vi "Main.vi"() -> ()   [LabVIEW 2020]
uses:
  <vilib>/Instr/_visa.llb/VISA Configure Serial Port (Instr).vi
panel:
  out "布尔":bool
  in  "帮助":bool
  in  "发送信息":bool
  in  "定时周期":dbl=1000.0 caption="周期："
  in  "发送新行":bool
  in  "定时发送":bool
  in  "发送信息":string
  in  "清除发送信息":bool
  in  "清除接收信息":bool
  out "接收信息":string
  out "状态指示灯":bool
  in  "串口操作":bool
  in  "停止位":u16(ring)=10 caption="停止位（10: 1位）" items=["1.0"=10, "1.5"=15, "2.0"=20]
  in  "数据位":u16(ring)=8 items=["8"=8, "7"=7, "6"=6, "5"=5]
  in  "检验位":enum16{"None", "Odd", "Even", "Mark", "Space"}(ring) caption="奇偶（0:无）"
  in  "波特率":u32(ring)=9600 items=["110"=110, "300"=300, "600"=600, "1200"=1200, "2400"=2400, "4800"=4800, "9600"=9600, "14400"=14400, "19200"=19200, "38400"=38400, "43000"=43000, "57600"=57600, "76800"=76800, "115200"=115200, "128000"=128000, "230400"=230400, "256000"=256000, "460800"=460800, "921600"=921600, "1000000"=1000000, "2000000"=2000000, "3000000"=3000000]
  in  "VISA资源名称":refnum<visa-resource-name>="COM1" caption="串口选择"
  in  "停止":bool
  # "ms"
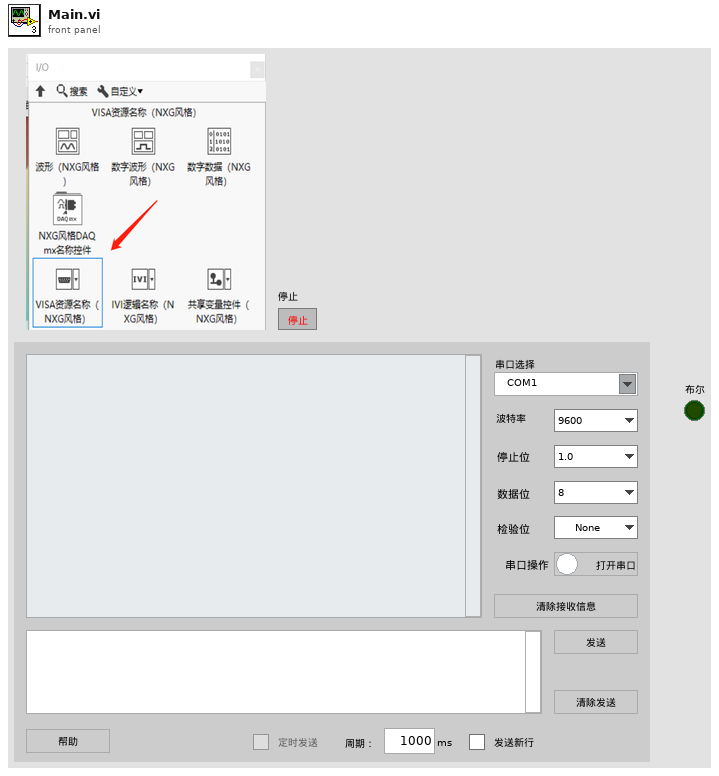
[diagram p1: front panel]
types:
  T1 = enum8{"Enabled", "Disabled", "Disabled and Grayed Out"}
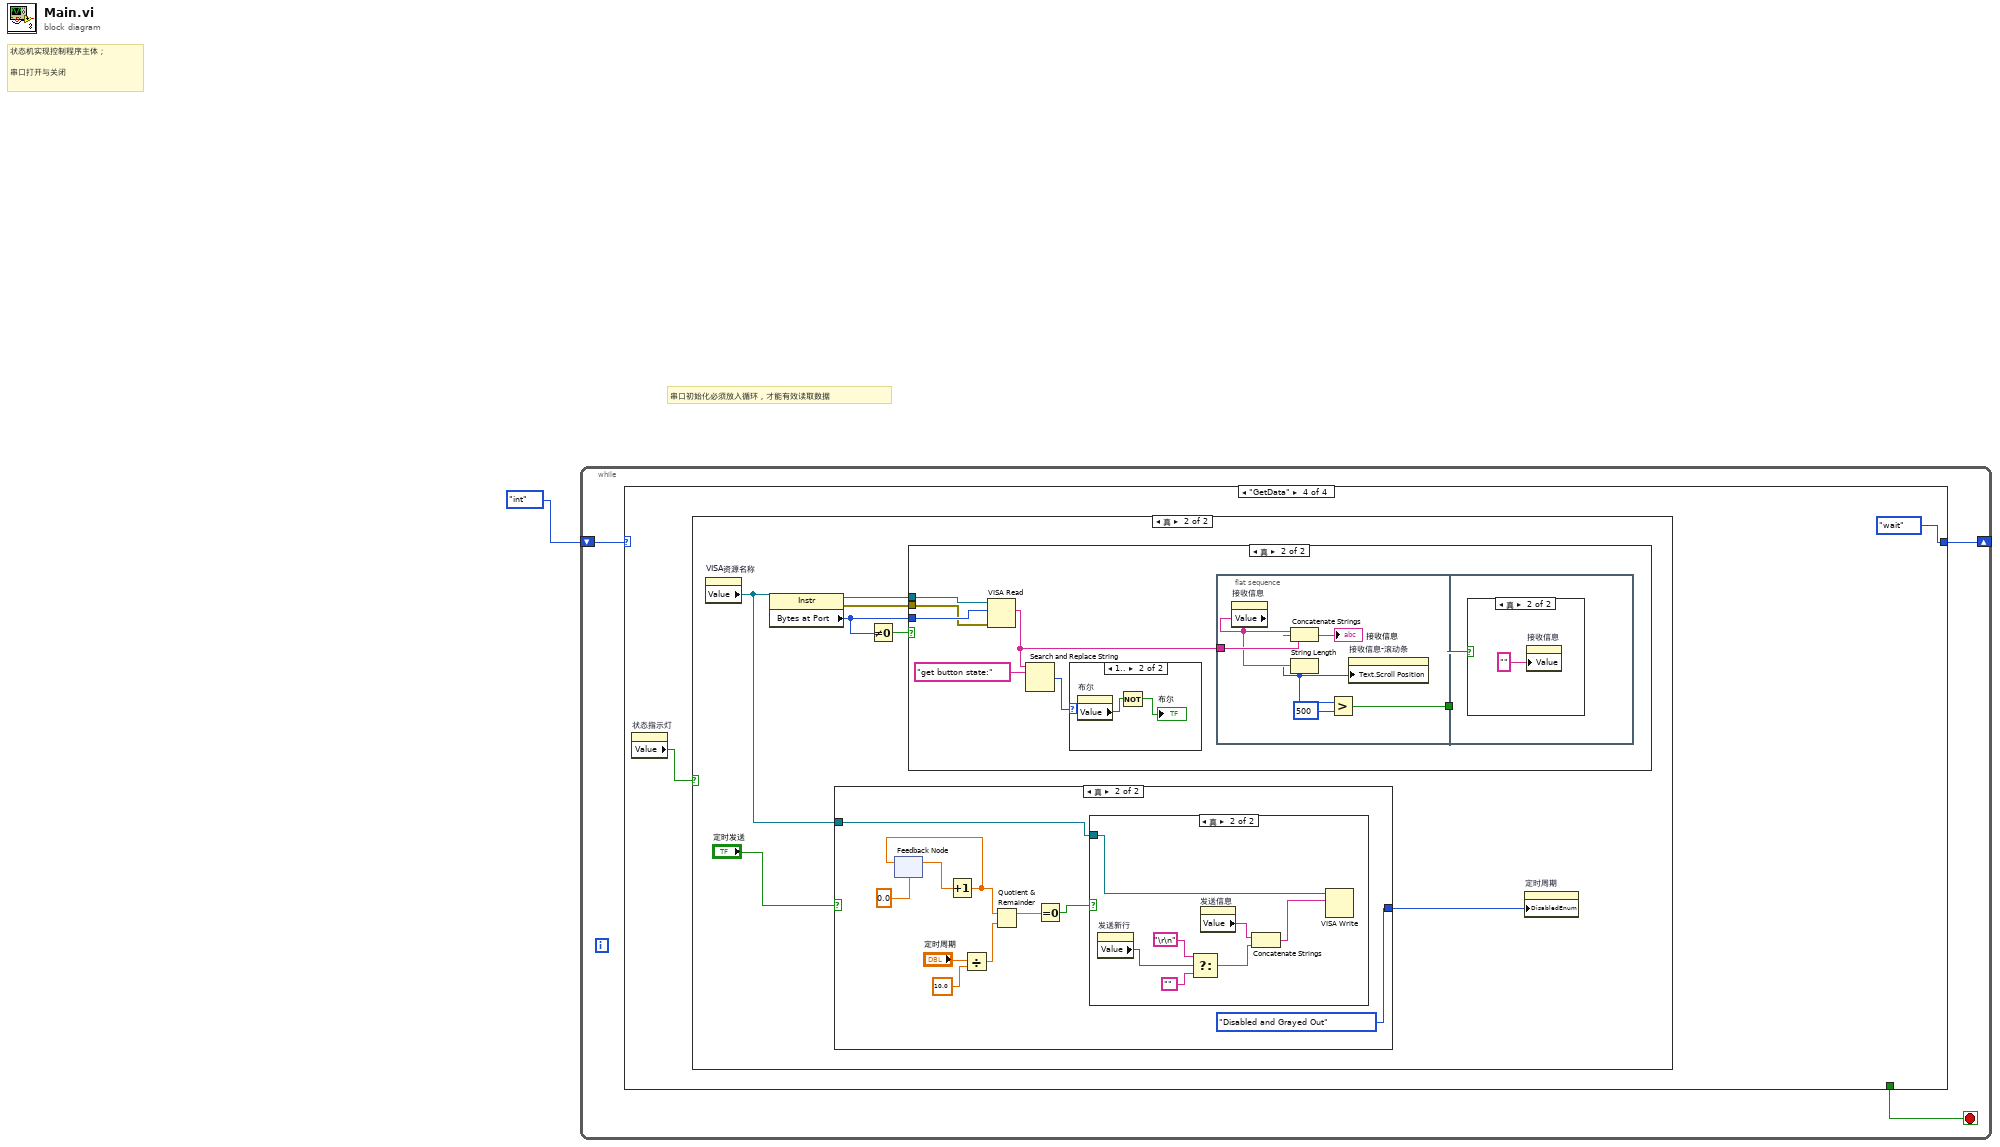
[diagram p0: block diagram]
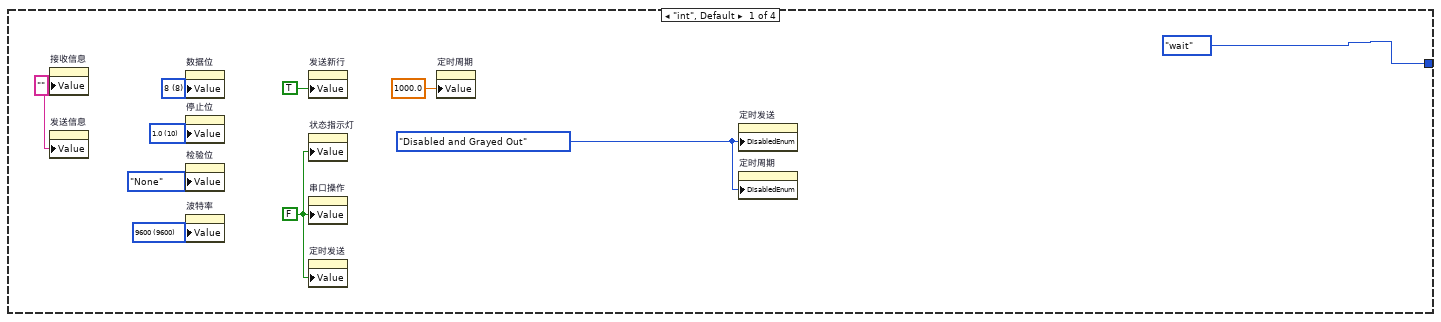
[diagram p2: hidden frame]
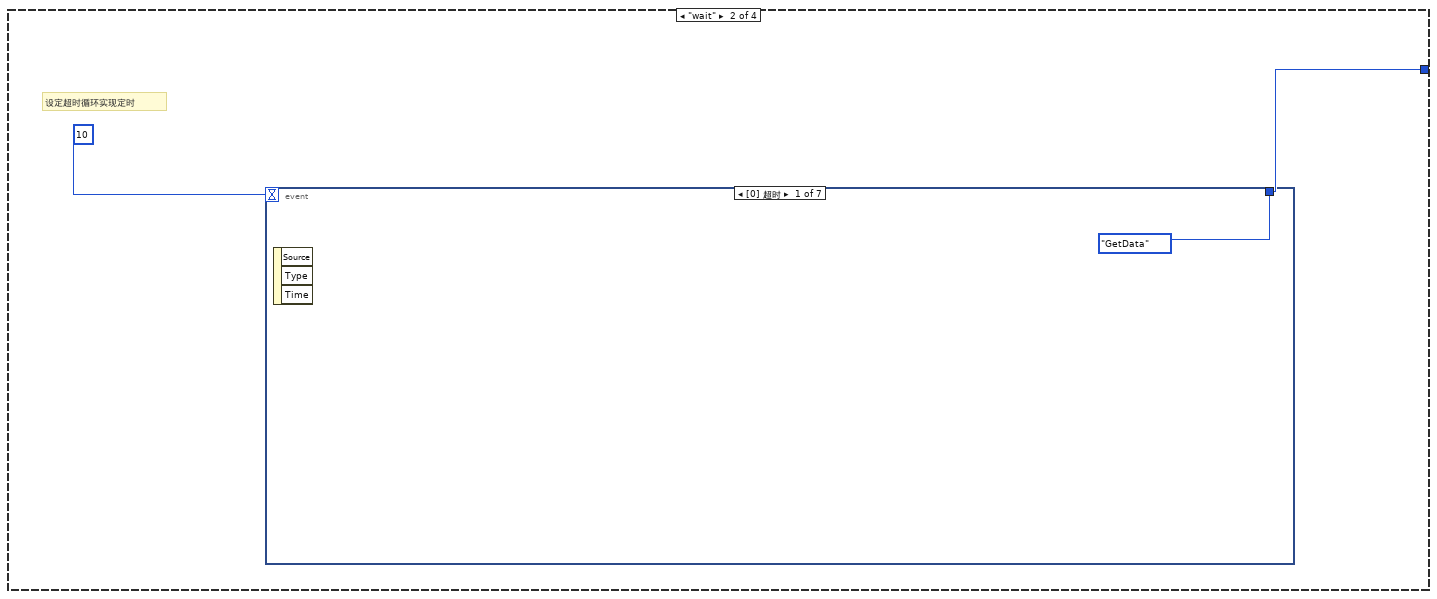
[diagram p3: hidden frame]
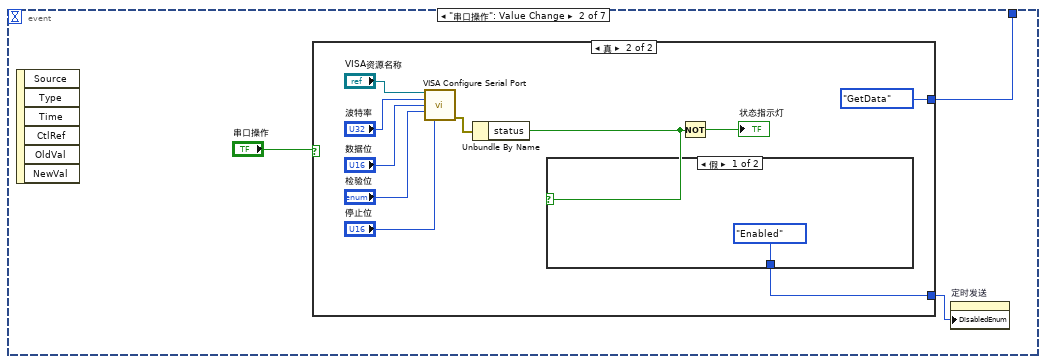
[diagram p4: hidden frame]
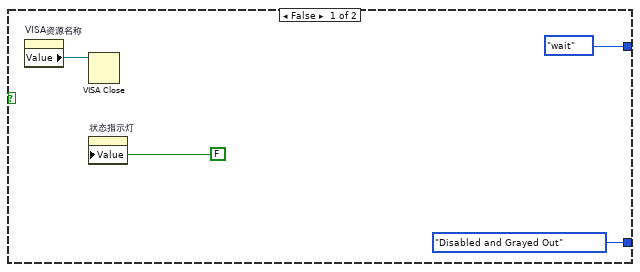
[diagram p5: hidden frame]
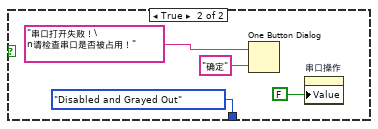
[diagram p6: hidden frame]
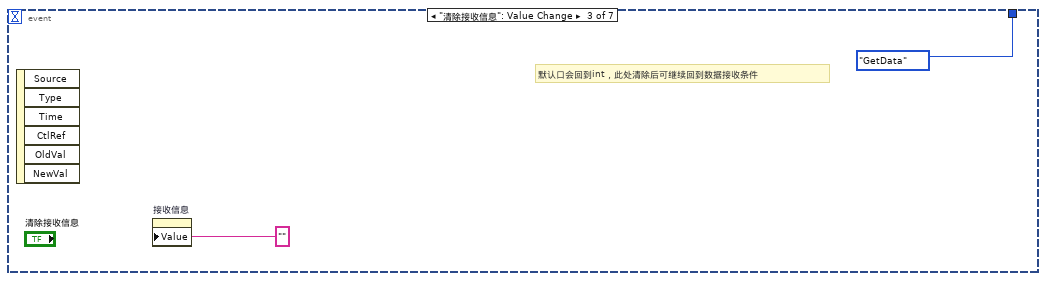
[diagram p7: hidden frame]
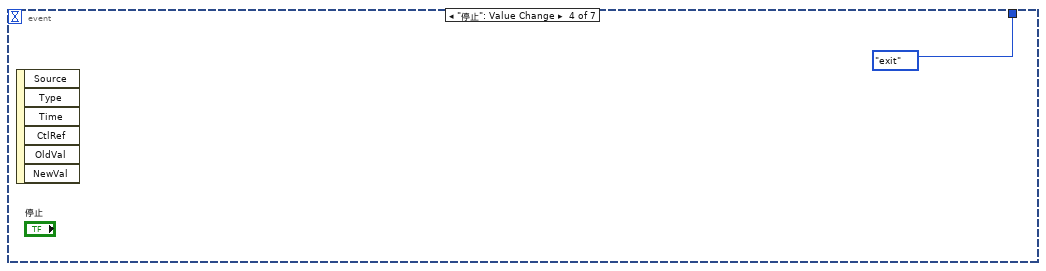
[diagram p8: hidden frame]
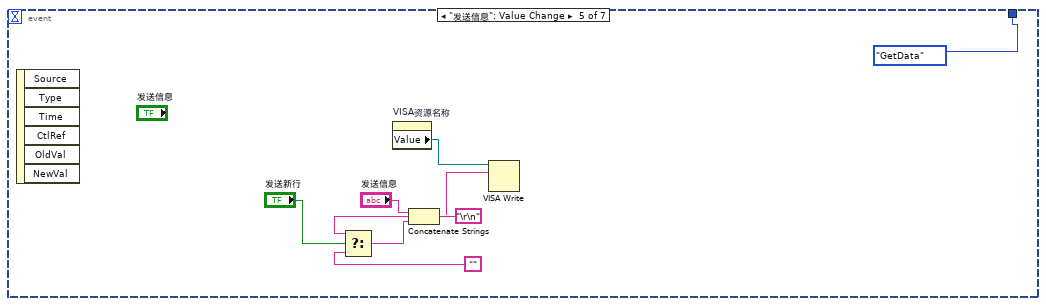
[diagram p9: hidden frame]
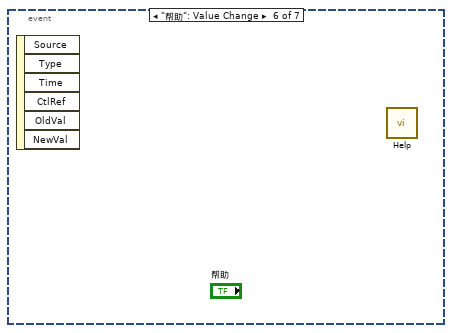
[diagram p10: hidden frame]
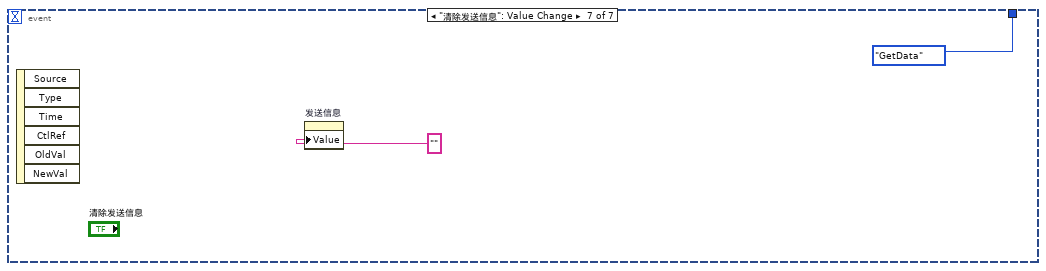
[diagram p11: hidden frame]
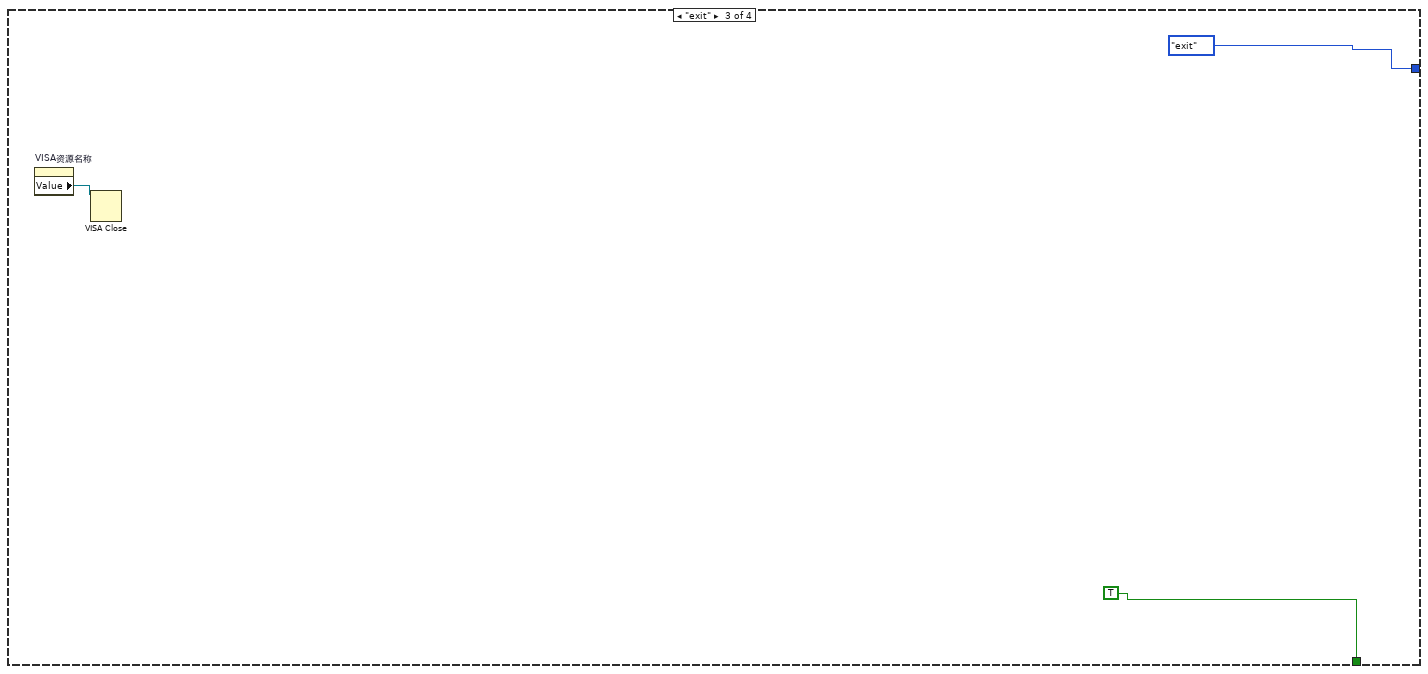
[diagram p12: hidden frame]
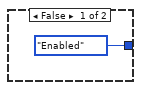
[diagram p14: hidden frame]
diagram:
  # "串口初始化必须放入循环，才能有效读取数据"
  # "状态机实现控制程序主体；\n\n串口打开与关闭"
  n1 = while {
    shift-right: [w3] -> _
    shift-left: enum16{"int", "wait", "exit", "GetData"}."int" -> [w4]
    stop <- w2 stop-if-true
    n2 = case shown="\"GetData\"" w4 {
      tunnel: [enum16{"int", "wait", "exit", "GetData"}."wait" w15 enum16{"int", "wait", "exit", "GetData"}."exit" enum16{"int", "wait", "exit", "GetData"}."wait"] -> w3
      tunnel: [_ _ TRUE _] -> w2
      frame "int", Default {
        w5 = T1."Disabled and Grayed Out" ("禁用")
        w6 = FALSE ("状态指示灯")
        w11 = u32 9600 items=["110"=110, "300"=300, "600"=600, "1200"=1200, "2400"=2400, "4800"=4800, "9600"=9600, "14400"=14400, "19200"=19200, "38400"=38400, "43000"=43000, "57600"=57600, "76800"=76800, "115200"=115200, "128000"=128000, "230400"=230400, "256000"=256000, "460800"=460800, "921600"=921600, "1000000"=1000000, "2000000"=2000000, "3000000"=3000000] ("波特率")
        w12 = u16 8 items=["8"=8, "7"=7, "6"=6, "5"=5] ("数据位")
        w13 = u16 10 items=["1.0"=10, "1.5"=15, "2.0"=20] ("停止位")
        w8 = "" ("接收信息")
        n3 = property on="接收信息" class="Str"("Value"=w8) -> ()  [unwired: 2 in, 2 out]
        n4 = property on="发送信息" class="Str"("Value"=w8) -> ()  [unwired: 2 in, 2 out]
        n5 = property on="数据位" class="Ring (严格)"("Value"=w12) -> ()  [unwired: 2 in, 2 out]
        n6 = property on="停止位" class="Ring (严格)"("Value"=w13) -> ()  [unwired: 2 in, 2 out]
        n7 = property on="检验位" class="Enum (严格)"("Value"=enum16{"None", "Odd", "Even", "Mark", "Space"}."None" ("检验位")) -> ()  [unwired: 2 in, 2 out]
        n8 = property on="波特率" class="Ring (严格)"("Value"=w11) -> ()  [unwired: 2 in, 2 out]
        n9 = property on="发送新行" class="Bool (严格)"("Value"=TRUE ("发送新行")) -> ()  [unwired: 2 in, 2 out]
        n10 = property on="状态指示灯" class="Bool (严格)"("Value"=w6) -> ()  [unwired: 2 in, 2 out]
        n11 = property on="串口操作" class="Bool (严格)"("Value"=w6) -> ()  [unwired: 2 in, 2 out]
        n12 = property on="定时发送" class="Bool (严格)"("Value"=w6) -> ()  [unwired: 2 in, 2 out]
        n13 = property on="定时周期" class="DigNum (严格)"("Value"=1000.0 ("定时周期")) -> ()  [unwired: 2 in, 2 out]
        n14 = property on="定时发送" class="Bool (严格)"("DisabledEnum"=w5) -> ()  [unwired: 2 in, 2 out]
        n15 = property on="定时周期" class="DigNum (严格)"("DisabledEnum"=w5) -> ()  [unwired: 2 in, 2 out]
      }
      frame "wait" {
        # "设定超时循环实现定时"
        n16 = event shown="[0] 超时" {
          selector: _ -> [_ _ _ _ _ _ _]
          dyn-events: _ -> [_ _ _ _ _ _ _]
          timeout: 10 -> [_ _ _ _ _ _ _]
          tunnel: [enum16{"int", "wait", "exit", "GetData"}."GetData" w19 enum16{"int", "wait", "exit", "GetData"}."GetData" enum16{"int", "wait", "exit", "GetData"}."exit" enum16{"int", "wait", "exit", "GetData"}."GetData" _ enum16{"int", "wait", "exit", "GetData"}."GetData"] -> w15
          event Timeout {
            n17 = event-data() -> ()  [unwired: 1 in, 3 out]
          }
          event "串口操作": Value Change {
            n18 = event-data() -> ()  [unwired: 1 in, 6 out]
            n19 = case shown="真" "串口操作" {
              tunnel: [enum16{"int", "wait", "exit", "GetData"}."wait" enum16{"int", "wait", "exit", "GetData"}."GetData"] -> w19
              tunnel: [T1."Disabled and Grayed Out" ("禁用") w25] -> w18
              frame False {
                n20 = property on="VISA资源名称" class="VISAName"() -> ("Value"=w23:refnum<visa-resource-name>)  [unwired: 2 in, 2 out]
                n21 = VISA Close(VISA resource name=w23) -> ()  [unwired: 1 in, 1 out]
                n22 = property on="状态指示灯" class="Bool (严格)"("Value"=FALSE ("状态指示灯")) -> ()  [unwired: 2 in, 2 out]
              }
              frame True {
                n23 = call-poly "VISA Configure Serial Port"("VISA resource name"="VISA资源名称", "baud rate (9600)"="波特率", "data bits (8)"="数据位", "parity (0:none)"="检验位", "stop bits (10: 1 bit)"="停止位") -> ("error out"=w29:errorcluster)  [unwired: 9 in, 1 out]
                n24 = Unbundle By Name(w29) -> ("status"=w26:bool)
                n25 = case shown="假" w26 {
                  tunnel: [T1."Enabled" ("禁用") T1."Disabled and Grayed Out" ("禁用")] -> w25
                  frame False {
                  }
                  frame True {
                    n26 = One Button Dialog(message="串口打开失败！\n请检查串口是否被占用！" ("消息"), button name ("OK")="确定" ("按钮名称（“确定”）")) -> ()  [unwired: 1 out]
                    n27 = property on="串口操作" class="Bool (严格)"("Value"=FALSE ("串口操作")) -> ()  [unwired: 2 in, 2 out]
                  }
                }
                n28 = Not(x=w26) -> (.not. x?=→"状态指示灯":bool)
              }
            }
            n29 = property on="定时发送" class="Bool (严格)"("DisabledEnum"=w18) -> ()  [unwired: 2 in, 2 out]
          }
          event "清除接收信息": Value Change {
            # "默认口会回到int，此处清除后可继续回到数据接收条件"
            n30 = event-data() -> ()  [unwired: 1 in, 6 out]
            n31 = property on="接收信息" class="Str"("Value"="" ("接收信息")) -> ()  [unwired: 2 in, 2 out]
          }
          event "停止": Value Change {
            n32 = event-data() -> ()  [unwired: 1 in, 6 out]
          }
          event "发送信息": Value Change {
            n33 = event-data() -> ()  [unwired: 1 in, 6 out]
            n34 = Select(t="\r\n", s="发送新行", f="") -> (s? t:f=w49:string)
            n35 = property on="VISA资源名称" class="VISAName"() -> ("Value"=w43:refnum<visa-resource-name>)  [unwired: 2 in, 2 out]
            n36 = Concatenate Strings("发送信息", w49) -> (w44:string)
            n37 = VISA Write(VISA resource name=w43, write buffer=w44) -> ()  [unwired: 1 in, 3 out]
          }
          event "帮助": Value Change {
            n38 = event-data() -> ()  [unwired: 1 in, 6 out]
            n39 = call "Help.vi"() -> ()  [unwired: 12 in]
          }
          event "清除发送信息": Value Change {
            n40 = event-data() -> ()  [unwired: 1 in, 6 out]
            n41 = property on="发送信息" class="Str"("Value"="" ("发送信息")) -> ()  [unwired: 2 in, 2 out]
          }
        }
      }
      frame "exit" {
        n42 = property on="VISA资源名称" class="VISAName"() -> ("Value"=w53:refnum<visa-resource-name>)  [unwired: 2 in, 2 out]
        n43 = VISA Close(VISA resource name=w53) -> ()  [unwired: 1 in, 1 out]
      }
      frame "GetData" {
        n44 = property on="状态指示灯" class="Bool (严格)"() -> ("Value"=w56:bool)  [unwired: 2 in, 2 out]
        n45 = case shown="真" w56 {
          frame False {
          }
          frame True {
            n46 = property on="VISA资源名称" class="VISAName"() -> ("Value"=w59:refnum<visa-resource-name>)  [unwired: 2 in, 2 out]
            n47 = property on="属性节点" class="Instr"(reference=w59) -> (reference out=w63:refnum<visa-resource-name>, error out=w62:errorcluster, "Bytes at Port"=w61:u32)  [unwired: 1 in]
            n48 = case shown="真" "定时发送" {
              tunnel: w59 -> [_ w67]
              tunnel: [T1."Enabled" ("禁用") T1."Disabled and Grayed Out" ("禁用")] -> w58
              frame False {
              }
              frame True {
                n49 = feedback #1(0.0) -> (w73:dbl)
                n50 = Increment(x=w73) -> (x+1=w69:dbl)
                n51 = feedback-in #1(w69) -> ()
                n52 = Divide(x="定时周期", y=10.0) -> (x/y=w74:dbl)
                n53 = Quotient & Remainder(x=w73, y=w74) -> (x-y*floor(x/y)=w75:dbl)  [unwired: 1 out]
                n54 = Equal To 0?(x=w75) -> (x = 0?=w68:bool)
                n55 = case shown="真" w68 {
                  tunnel: w67 -> [_ w76]
                  frame False {
                  }
                  frame True {
                    n56 = property on="发送新行" class="Bool (严格)"() -> ("Value"=w81:bool)  [unwired: 2 in, 2 out]
                    n57 = Select(t="\r\n", s=w81, f="") -> (s? t:f=w80:string)
                    n58 = property on="发送信息" class="Str"() -> ("Value"=w82:string)  [unwired: 2 in, 2 out]
                    n59 = Concatenate Strings(w82, w80) -> (w79:string)
                    n60 = VISA Write(VISA resource name=w76, write buffer=w79) -> ()  [unwired: 1 in, 3 out]
                  }
                }
              }
            }
            n61 = Not Equal To 0?(x=w61) -> (x != 0?=w64:bool)
            n62 = case shown="真" w64 {
              tunnel: w63 -> [_ w88]
              tunnel: w62 -> [_ w87]
              tunnel: w61 -> [_ w89]
              frame False {
              }
              frame True {
                n63 = VISA Read(VISA resource name=w88, byte count=w89, error in (no error)=w87) -> (read buffer=w85:string)  [unwired: 3 out]
                n64 = Search and Replace String(input string=w85, search string="get button state:" ("搜索字符串")) -> (number of replacements=w83:i32)  [unwired: 6 in, 3 out]
                n65 = case shown="1.." w83 {
                  frame 0, Default {
                  }
                  frame 1.. {
                    n66 = property on="布尔" class="Bool (严格)"() -> ("Value"=w91:bool)  [unwired: 2 in, 2 out]
                    n67 = Not(x=w91) -> (.not. x?=→"布尔":bool)
                  }
                }
                n68 = flat-sequence {
                  tunnel: w85 -> [w97]
                  tunnel: [w92] -> w86
                  tunnel: w86 -> [w98]
                  frame #0 {
                    n69 = property on="接收信息" class="Str"() -> ("Value"=w95:string)  [unwired: 2 in, 2 out]
                    n70 = Concatenate Strings(w95, w97) -> (→"接收信息":string)
                    n71 = String Length(string=w95) -> (length=w93:i32)
                    n72 = Greater?(x=w93, y=500) -> (0:w92:bool)
                    n73 = property on="接收信息-滚动条" class="Str"("Text.Scroll Position"=w93) -> ()  [unwired: 2 in, 2 out]
                  }
                  frame #1 {
                    n74 = case shown="真" w98 {
                      frame False {
                      }
                      frame True {
                        n75 = property on="接收信息" class="Str"("Value"="" ("接收信息")) -> ()  [unwired: 2 in, 2 out]
                      }
                    }
                  }
                }
              }
            }
            n76 = property on="定时周期" class="DigNum (严格)"("DisabledEnum"=w58) -> ()  [unwired: 2 in, 2 out]
          }
        }
      }
    }
  }
